vi "Conductus Write Heater Power.vi"(1 "Setpoint":dbl min=0.0 max=100.0 step=0.001 format="%.3f", 2 "Instrument Address":refnum<visa-resource-name>) -> ()   [LabVIEW 2021]
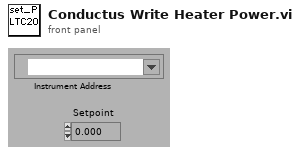
[diagram p1: front panel]
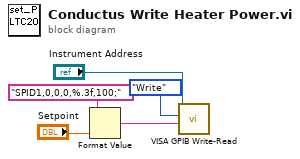
[diagram p0: block diagram]
diagram:
  n1 = Format Value(format string="SPID1,0,0,0,%.3f,100;", value (0)="Setpoint") -> (output string=w2:string)  [unwired: 1 in]
  n2 = call "VISA GPIB Write-Read.vi"("Command"=w2, "Action"=enum16{"Write", "Read", "Write & Read"}."Write", "VISA resource name"="Instrument Address") -> ()  [unwired: 5 in, 4 out]
